vi "util_get_filename.vi"(8 "error in (no error)":errorcluster, 11 "filename_with_extension":string) -> (0 "error out":errorcluster, 3 "filename_without_extension":string)   [LabVIEW 2015, in "lv-bin-7zip.lvlib"]
uses:
  lv-bin-7zip.lvlib
  <userlib>/antonio-alexander/lv-bin/public/api/v1/v1.lvlib
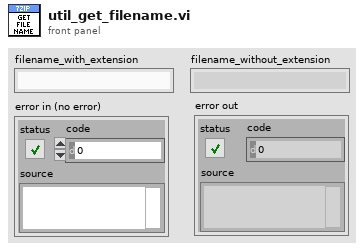
[diagram p1: front panel]
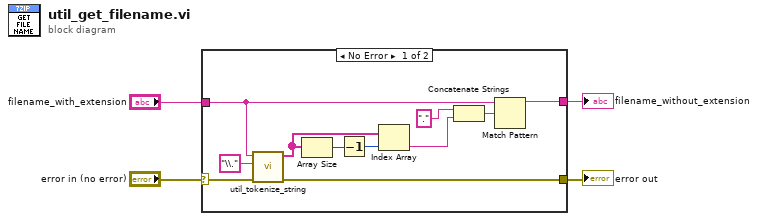
[diagram p0: block diagram]
diagram:
  n1 = case shown="No Error" "error in (no error)" {
    selector: "error in (no error)" -> [w6 w16]
    tunnel: [w15 _] -> w4
    tunnel: "filename_with_extension" -> [w9 _]
    tunnel: [w5 w16] -> w1
    frame No Error {
      n2 = call <userlib>:"util_tokenize_string.vi"("error in (no error)"=w6, "delimiter"="\\." ("delimiter ([\\s\\t\\n\\r]+)"), "input_string"=w9) -> ("error out"=w5:errorcluster, "before_match []"=w7:string[])  [unwired: 6 in, 1 out]
      n3 = Array Size(array=w7) -> (size(s)=w14:i32)
      n4 = Decrement(x=w14) -> (x-1=w13:i32)
      n5 = Index Array(array=w7, index=w13) -> (element=w12:string)
      n6 = Concatenate Strings("." ("string"), w12) -> (w10:string)
      n7 = Match Pattern(string=w9, regular expression=w10) -> (before substring=w15:string)  [unwired: 1 in, 3 out]
    }
    frame Error {
    }
  }
  "filename_without_extension" <- w4
  "error out" <- w1
